vi "Test Prop.vi"() -> ()   [LabVIEW 2020, in "Rover.lvlib" / "Rover.lvclass"]
uses:
  Rover.lvclass
  Pose.ctl
  <vilib>/MakerHub/LINX/Public/Utilities/Open Local.vi
  <vilib>/MakerHub/LINX/LMH-LINX.lvlib
panel:
  out "Pose":T1
  out "error out":errorcluster
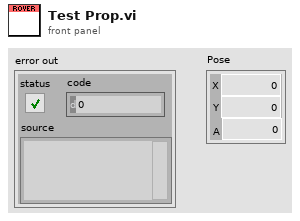
[diagram p1: front panel]
types:
  T1 = typedef "Rover.lvlib/Rover.lvclass/Pose.ctl" = cluster{"X":sgl, "Y":sgl, "A":sgl}
  T2 = typedef "LMH-LINX.lvlib/LINX Ref.ctl" = cluster{"IO":T3, "Interface":T4, "LINX Device Config":T5}
  T3 = typedef "LMH-LINX.lvlib/Platform.ctl" = enum16{"Remote", "Local"}
  T4 = typedef "LMH-LINX.lvlib/Interface.ctl" = enum16{"Serial", "TCP"}
  T5 = typedef "LMH-LINX.lvlib/Device.lvlib/LINX Device Config.ctl" = cluster{"Interface":T4, "COM Port":refnum<visa-resource-name>, "TCP Configuration":T6, "Device Family":u8, "Device ID":u8, "Device Name":string, "TCP Ref":refnum<k5>, "Channels":T7}
  T6 = typedef "LMH-LINX.lvlib/Device.lvlib/TCP Config.ctl" = cluster{"IP Address":string, "Port":u16}
  T7 = typedef "LMH-LINX.lvlib/Channels.ctl" = cluster{"DI":u8[], "DO":u8[], "AI":u8[], "AO":u8[], "PWM":u8[], "QE":u8[], "UART":u8[], "I2C 2":u8[], "SPI":u8[], "CAN":u8[], "Servo":u8[], "AI Ref (V)":dbl, "AI Resolution (Bits)":u8, "AO Ref (V)":dbl, "AO Resolution (Bits)":u8}
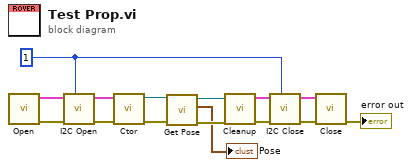
[diagram p0: block diagram]
diagram:
  w6 = u8 1 ("I2C Channel (0)")
  n1 = call-poly <vilib>:"Open.vi"() -> ("Error Out"=w14:errorcluster, "LINX Resource"=w15:T2)  [unwired: 9 in, 1 out]
  n2 = call <vilib>:"I2C Open.vi"("I2C Channel (0)"=w6, "Error In"=w14, "LINX Resource"=w15) -> ("Error Out"=w12:errorcluster, "LINX Resource"=w13:T2)  [unwired: 7 in]
  n3 = call "Ctor.vi"("error in (no error)"=w12, "LINX Resource"=w13) -> ("error out"=w4:errorcluster, "Rover out"=w5:refnum<class "Rover.lvclass">)  [unwired: 8 in]
  n4 = call "Get Pose.vi"("error in (no error)"=w4, "Rover in"=w5) -> ("error out"=w3:errorcluster, "Pose"=→"Pose":T1, "Rover out"=w2:refnum<class "Rover.lvclass">)  [unwired: 7 in]
  n5 = call "Cleanup.vi"("error in (no error)"=w3, "Rover in"=w2) -> ("error out"=w7:errorcluster, "LINX Resource"=w8:T2)  [unwired: 8 in]
  n6 = call <vilib>:"I2C Close.vi"("I2C Channel (0)"=w6, "Error In"=w7, "LINX Resource"=w8) -> ("Error Out"=w10:errorcluster, "LINX Resource"=w11:T2)  [unwired: 7 in]
  n7 = call <vilib>:"Close.vi"("Error In"=w10, "LINX Resource"=w11) -> ("Error Out"=→"error out":errorcluster)  [unwired: 9 in]
